vi "Análise de dados Json Forno.vi"() -> ()   [LabVIEW 2021]
panel:
  out "Temperatura":dbl(graph)
  out "Energia":dbl(graph)
  out "Potência":dbl(graph)
  out "Corrente":dbl(graph)
  out "Tensão":dbl(graph)
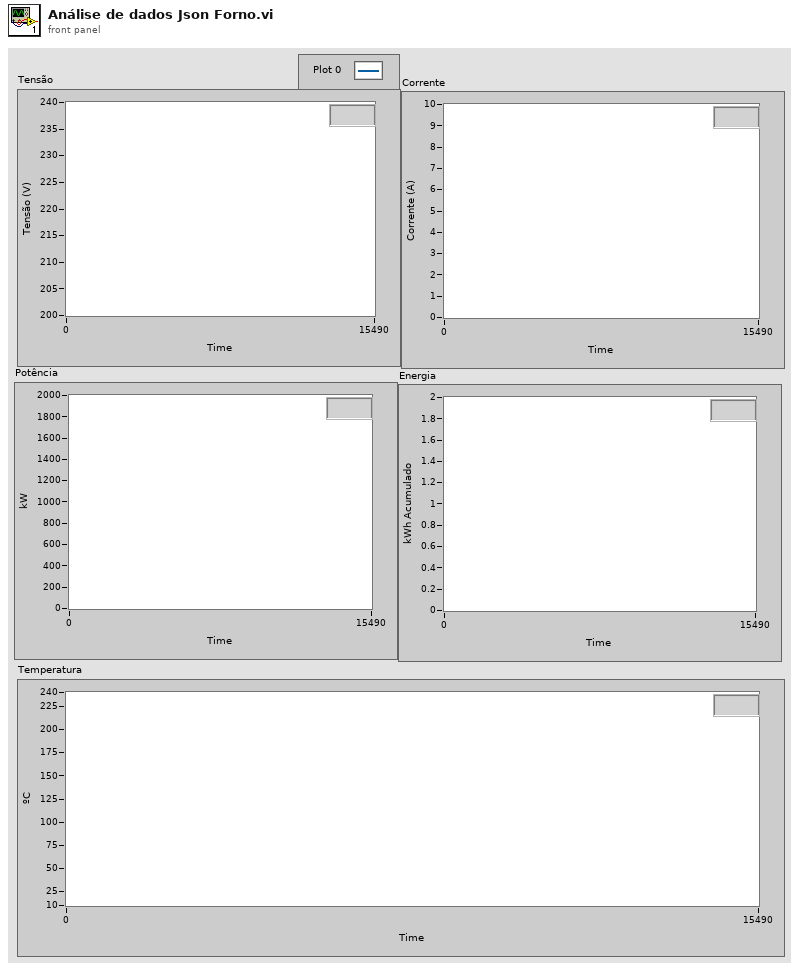
[diagram p1: front panel]
types:
  T1 = cluster{"Tensao":dbl, "Corrente":dbl, "Potencia":dbl, "Energia":dbl, "Temperatura":dbl}
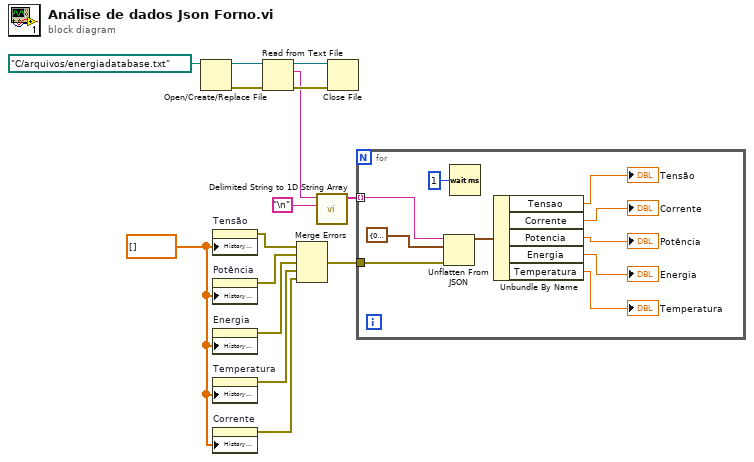
[diagram p0: block diagram]
diagram:
  w7 = dbl[] [] ("History Data")
  n1 = Open/Create/Replace File(file path (use dialog)=path "C:/arquivos/energiadatabase.txt") -> (refnum out=w15:refnum<file>, error out=w14:errorcluster)  [unwired: 5 in, 1 out]
  n2 = property on="Tensão" class="WFChart (strict)"("History Data"=w7) -> (error out=w6:errorcluster)  [unwired: 2 in, 1 out]
  n3 = property on="Potência" class="WFChart (strict)"("History Data"=w7) -> (error out=w5:errorcluster)  [unwired: 2 in, 1 out]
  n4 = property on="Energia" class="WFChart (strict)"("History Data"=w7) -> (error out=w4:errorcluster)  [unwired: 2 in, 1 out]
  n5 = property on="Temperatura" class="WFChart (strict)"("History Data"=w7) -> (error out=w3:errorcluster)  [unwired: 2 in, 1 out]
  n6 = property on="Corrente" class="WFChart (strict)"("History Data"=w7) -> (error out=w2:errorcluster)  [unwired: 2 in, 1 out]
  n7 = Read from Text File(file (use dialog)=w15, error in=w14) -> (refnum out=w13:refnum<file>, text=w10:string, error out=w12:errorcluster)  [unwired: 2 in, 1 out]
  n8 = Merge Errors(w6, w5, w4, w3, w2) -> (w1:errorcluster)
  n9 = call <vilib>:"Delimited String to 1D String Array.vi"("delimiter"="\n", "delimited string"=w10) -> ("string array"=w8:string[])  [unwired: 9 in]
  n10 = Close File(refnum=w13, error in=w12) -> ()  [unwired: 2 out]
  n11 = for {
    tunnel: w8 -> [w25] mode=indexing
    tunnel: w1 -> [w24]
    n12 = Unflatten From JSON(JSON string=w25, type and defaults=T1 {"Tensao"=0.0, "Corrente"=0.0, "Potencia"=0.0, "Energia"=0.0, "Temperatura"=0.0}, error in (no error)=w24) -> (value=w22:T1)  [unwired: 4 in, 1 out]
    n13 = Wait (ms)(milliseconds to wait=u32 1) -> ()  [unwired: 1 out]
    n14 = Unbundle By Name(w22) -> ("Tensao"=→"Tensão":dbl, "Corrente"=→"Corrente":dbl, "Potencia"=→"Potência":dbl, "Energia"=→"Energia":dbl, "Temperatura"=→"Temperatura":dbl)
  }
